vi "NewTemplate.Init.vi"(6 "JQMHStartup in":refnum<class "RQMHStartup.lvclass">, 8 "error in (no error)":errorcluster, 11 "NewTemplate in":refnum<class "SingleLoopTemplate.lvclass">) -> (0 "error out":errorcluster, 1 "StartupParams":variant, 2 "Requests":T2, 3 "NewTemplate out":refnum<class "SingleLoopTemplate.lvclass">, 4 "JQMHStartup out":refnum<class "RQMHStartup.lvclass">, 5 "StandardRequests":refnum<event-registration>, 7 "External Start?":bool)   [LabVIEW 2025, in "SingleLoopTemplate.lvclass"]
uses:
  SingleLoopTemplate.lvclass
  RQMHCore/Startup/RQMHStartup.lvclass
  RQMHCore/ModuleCore/StopEventArgs.ctl
  Request Events--cluster.ctl
  Do Something Args.ctl
  RQMHCore/ModuleCore/Reply.ctl
  RQMHCore/ModuleCore/StandardRequests.ctl
  RQMHCore/ModuleCore/InitialiseArgs.ctl
  RQMHCore/ModuleCore/Show Front Panel--Args.ctl
  RQMHCore/ModuleCore/Hide Front Panel.ctl
  RQMHCore/ModuleCore/Show Block Diagram.ctl
  RQMHCore/ModuleCore/Hide Block Diagram--Args.ctl
  RQMHCore/ModuleCore/RQMHModule.lvclass/RQMHModule.ctl
  SingleLoopTemplate.lvclass/SingleLoopTemplate.ctl
  C:/Git/JA/JQMH/RQMHCore/ModuleCore/RQMHModule.lvclass
  RQMHCore/Shared/RQMHShared.lvlib
  RQMHCore/ModuleCore/RQMHModule.lvclass
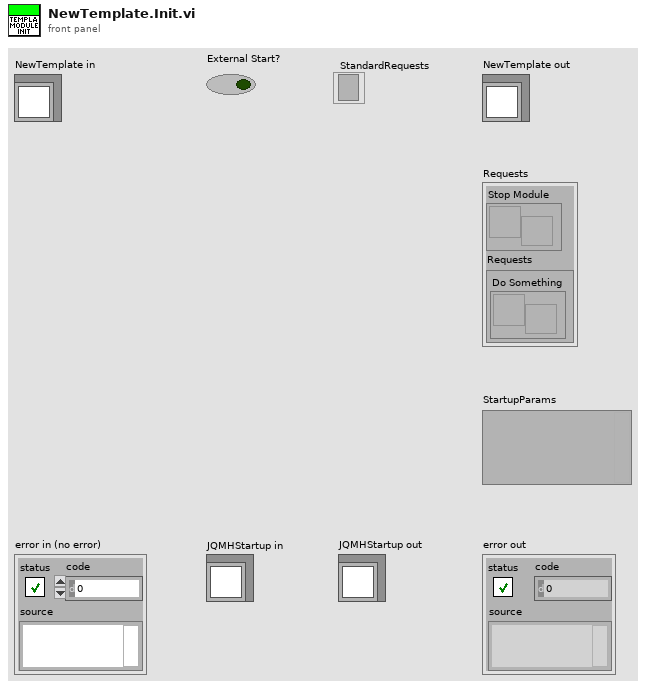
[diagram p1: front panel]
types:
  T1 = typedef "SingleLoopTemplate.lvclass/Request Events--cluster.ctl" = cluster{"Do Something":refnum<user-event>}
  T2 = cluster{"Stop Module":refnum<user-event>, "Requests":T1}
  T3 = typedef "RQMHModule.lvclass/StandardRequests.ctl" = cluster{"Initialise":refnum<user-event>, "Stop Module":refnum<user-event>, "ShowFP":refnum<user-event>, "Hide Front Panel":refnum<user-event>, "Show Block Diagram":refnum<user-event>, "Hide Block Diagram":refnum<user-event>}
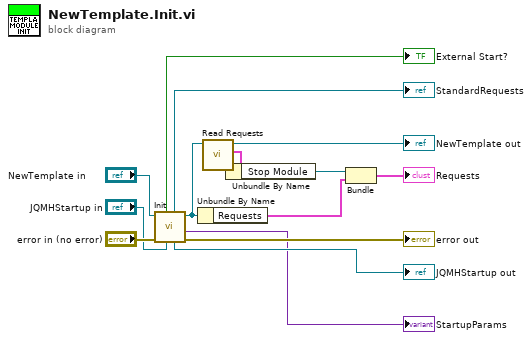
[diagram p0: block diagram]
diagram:
  n1 = call "Init.vi"("JQMHStartup.lvclass"="JQMHStartup in", "error in (no error)"="error in (no error)", "JQMHCore.lvclass"="NewTemplate in") -> ("error out"=→"error out":errorcluster, "StartupParams"=→"StartupParams":variant, "JQMHCore out"=w13:refnum<class "SingleLoopTemplate.lvclass">, "JQMHStartup out"=→"JQMHStartup out":refnum<class "RQMHStartup.lvclass">, "Event Registration Refnum"=→"StandardRequests":refnum<event-registration>, "External Start?"=→"External Start?":bool)  [unwired: 3 in]
  n2 = Unbundle By Name(w13) -> ("Requests"=w14:T1)
  n3 = call "Read Requests.vi"("JQMHModule in"=w13) -> ("Requests"=w6:T3, "JQMHModule out"=→"NewTemplate out":refnum<class "SingleLoopTemplate.lvclass">)  [unwired: 9 in]
  n4 = Unbundle By Name(w6) -> ("Stop Module"=w5:refnum<user-event>)
  n5 = Bundle("Stop Module"=w5, "Requests"=w14) -> (→"Requests":T2)  [unwired: 1 in]
